vi "WriteRowU8.vi"(8 "error in":errorcluster, 9 "Pixel Row":u8[](array[numeric]), 10 "Row":i32, 11 "Image Reference In":T1) -> (0 "error out":errorcluster, 3 "Image Reference Out":T1)   [LabVIEW 2020, in "OpenLvVision_Image.lvlib" / "DataAccess.lvlib"]
doc: "Write all pixel values in an row."
uses:
  DataAccess.lvlib
  Management/TypeDef/Image.ctl
  <vilib>/Utility/error.llb/Error Cluster From Error Code.vi
  <vilib>/ErrorRing/Error Ring.xnode
  Management/Management.lvlib
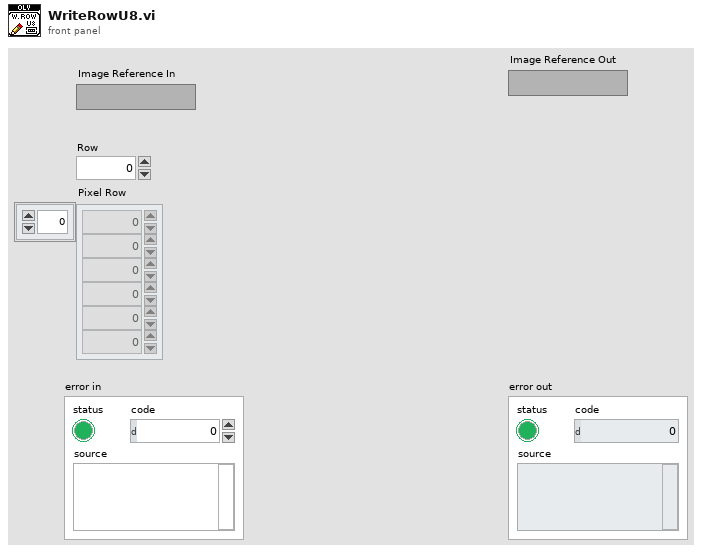
[diagram p1: front panel]
types:
  T1 = typedef "OpenLvVision_Image.lvlib/Management.lvlib/Image.ctl" = refnum<image>
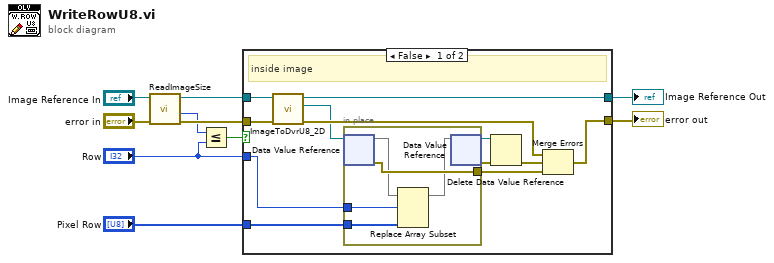
[diagram p0: block diagram]
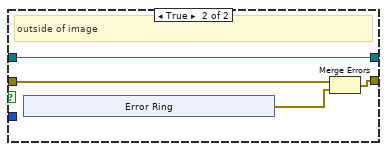
[diagram p2: hidden frame]
diagram:
  n1 = call "ReadImageSize.vi"("error in"="error in", "Image Reference In"="Image Reference In") -> ("error out"=w9:errorcluster, "Height"=w2:i32, "Image Reference Out"=w10:T1)  [unwired: 6 in, 1 out]
  n2 = Less Or Equal?(x=w2, y="Row") -> (x <= y?=w4:bool)
  n3 = case shown="False" w4 {
    tunnel: w10 -> [w22 w29]
    tunnel: w9 -> [w21 w31]
    tunnel: [w20 w29] -> w6
    tunnel: [w13 w28] -> w5
    tunnel: "Row" -> [w12 _]
    tunnel: "Pixel Row" -> [w11 _]
    frame False {
      # "inside image"
      n4 = call "ImageToDvrU8_2D.vi"("error in"=w21, "Image Reference In"=w22) -> ("error out"=w15:errorcluster, "EDVR 2D U8"=w14:refnum<data-value>, "Image Reference Out"=w20:T1)  [unwired: 6 in, 1 out]
      n5 = in-place {
        in-place-border: [w27] -> w18
        in-place-border: w12 -> [w24]
        in-place-border: w11 -> [w23]
        n6 = in-place-dvr #1(w14) -> (w26:u8[][], w27:errorcluster)
        n7 = Replace Array Subset(array=w26, new element=w23, index (row)=w24) -> (w25:u8[][])  [unwired: 1 in]
        n8 = in-place-dvr #1(w25) -> (w16:refnum<data-value>, w17:errorcluster)
      }
      n9 = Delete Data Value Reference(data value reference=w16, error in=w17) -> (error out=w19:errorcluster)  [unwired: 1 out]
      n10 = Merge Errors(w15, w19, w18) -> (w13:errorcluster)
    }
    frame True {
      # "outside of image"
      n11 = xnode "Error Ring"() -> ("error out"=w30:errorcluster)
      n12 = Merge Errors(w31, w30) -> (w28:errorcluster)
    }
  }
  "error out" <- w5
  "Image Reference Out" <- w6
